vi "LV_n_UDP_clients.vi"() -> ()   [LabVIEW 2020]
panel:
  out "2nd port":string
  out "1st port":string
  in  "Open Multi Ports":bool
  in  "Open Single Port":bool
  in  "Send Test Image":bool
  in  "h":i32=10 min=1 max=5000 step=1
  in  "w":i32=1 min=1 max=5000 step=1
  out "Elaps ms":u32
  in  "Send Image":bool
  out "Path to Python script":path
  in  "Stop":bool
  out "Answer":string
  in  "Ping":bool
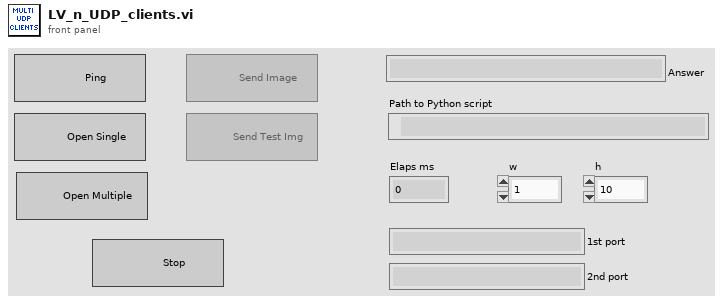
[diagram p1: front panel]
types:
  T1 = enum8{"Enabled", "Disabled", "Disabled and Grayed Out"}
  T2 = typedef "Image Type" = u32
  T3 = typedef "IMAQ Image.ctl" = refnum<image>
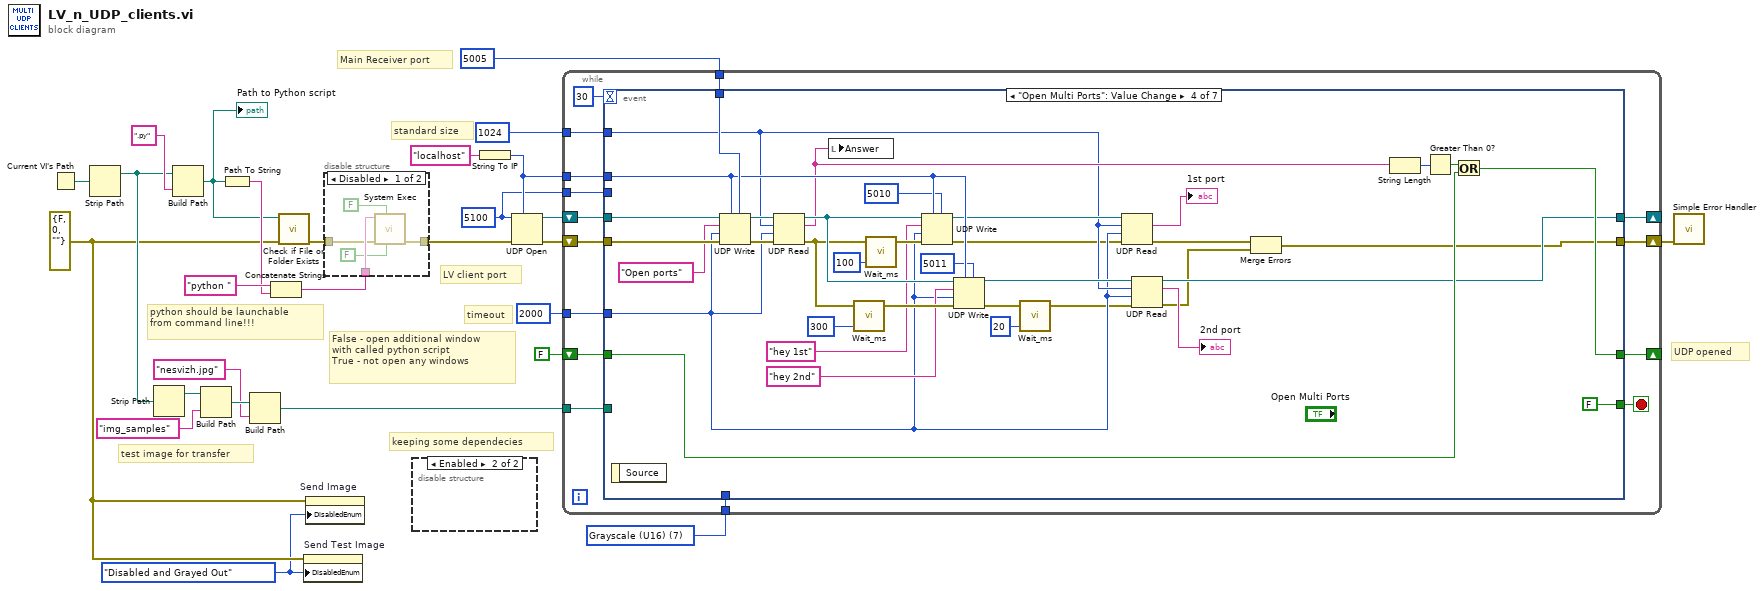
[diagram p0: block diagram]
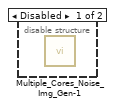
[diagram p2: hidden frame]
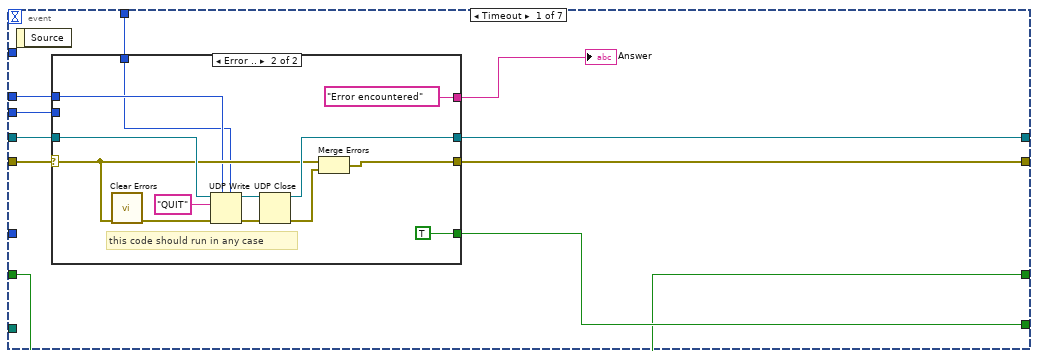
[diagram p4: hidden frame]
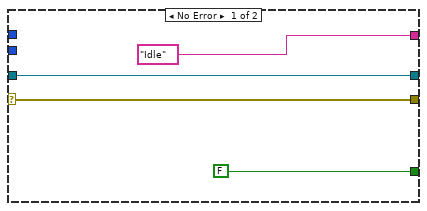
[diagram p5: hidden frame]
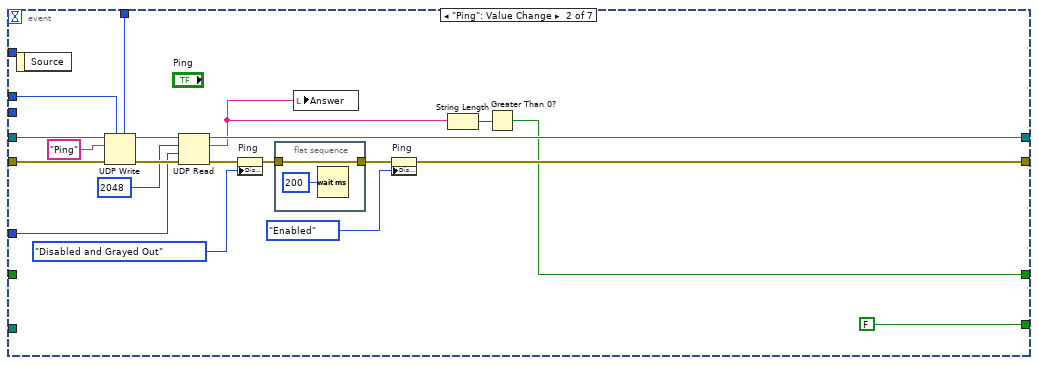
[diagram p6: hidden frame]
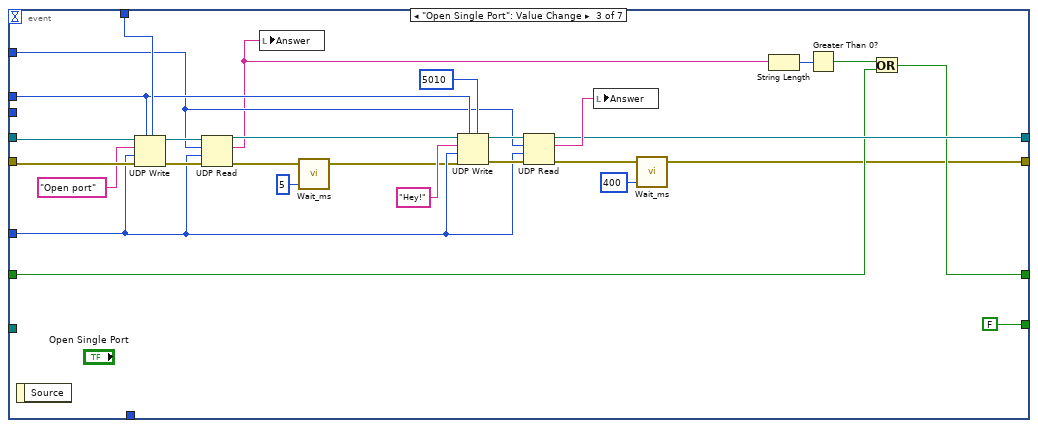
[diagram p7: hidden frame]
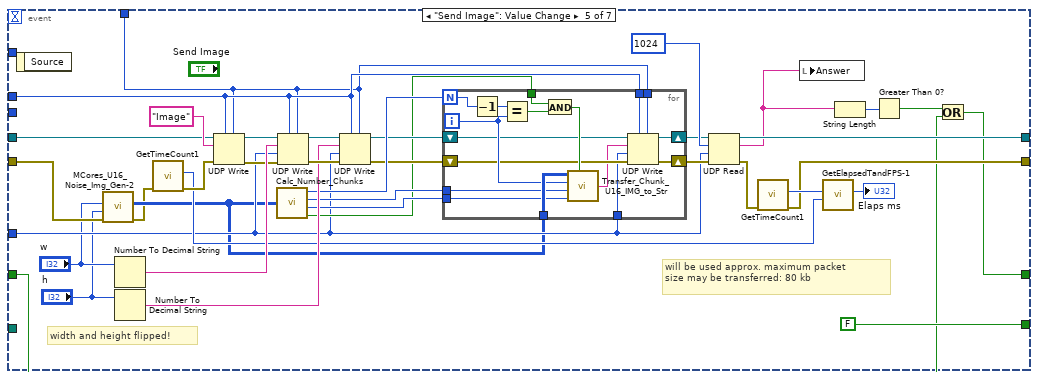
[diagram p8: hidden frame]
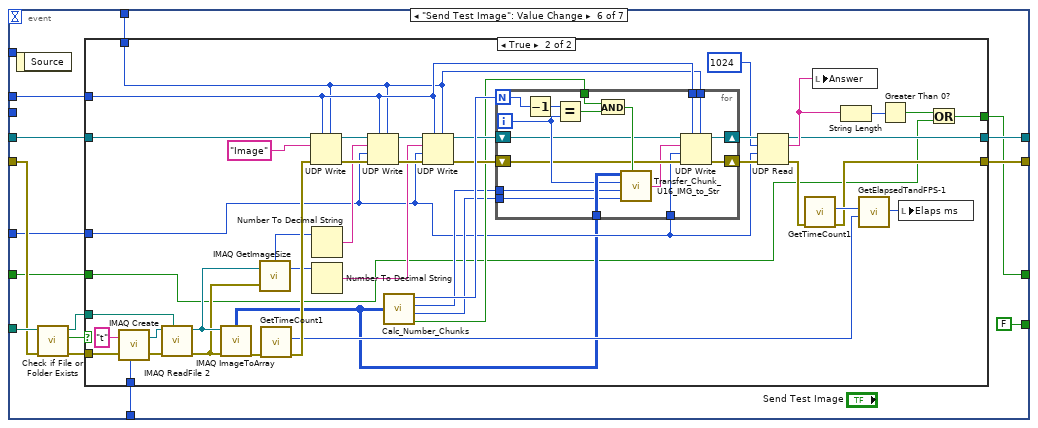
[diagram p9: hidden frame]
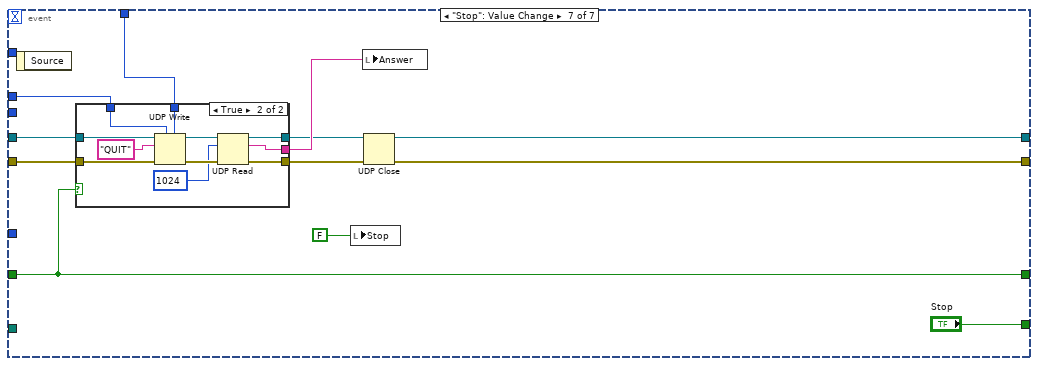
[diagram p11: hidden frame]
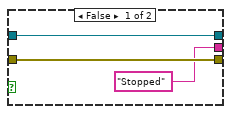
[diagram p12: hidden frame]
diagram:
  w3 = T1."Disabled and Grayed Out" ("Disabled")
  w5 = T2 7 items=["Grayscale (U8)", "Grayscale (I16)", "Grayscale (SGL)", "Complex (CSG)", "RGB (U32)", "HSL (U32)", "RGB (U64)", "Grayscale (U16)"] ("Image Type")
  w14 = u16 5100 ("remote port or service name")
  w4 = errorcluster {"status"=FALSE, "code"=0, "source"=""} ("error in (no error)")
  # "standard size"
  # "UDP opened"
  # "test image for transfer"
  # "keeping some dependecies"
  # "timeout"
  # "Main Receiver port"
  # "LV client port"
  # "False - open additional window\nwith called python script\nTrue - not open any windows"
  # "python should be launchable \nfrom command line!!!"
  n1 = Current VI's Path() -> (path=w26:path)
  n2 = Strip Path(path=w26) -> (stripped path=w11:path)  [unwired: 1 out]
  n3 = Strip Path(path=w11) -> (stripped path=w10:path)  [unwired: 1 out]
  n4 = Build Path(base path=w11, name or relative path=".py" ("string")) -> (appended path=w21:path)
  "Path to Python script" <- w21
  n5 = Build Path(base path=w10, name or relative path="img_samples" ("string")) -> (appended path=w8:path)
  n6 = Path To String(path=w21) -> (string=w22:string)
  n7 = Build Path(base path=w8, name or relative path="nesvizh.jpg" ("string")) -> (appended path=w6:path)
  n8 = Concatenate Strings("python " ("command line"), w22) -> (w24:string)
  n9 = call <vilib>:"Check if File or Folder Exists.vi"("error in (no error)"=w4, "path"=w21) -> ("error out"=w20:errorcluster)  [unwired: 7 in, 2 out]
  n10 = property on="Send Test Image" class="Bool"(error in=w4, "DisabledEnum"=w3) -> ()  [unwired: 1 in, 2 out]
  n11 = property on="Send Image" class="Bool"(error in=w4, "DisabledEnum"=w3) -> ()  [unwired: 1 in, 2 out]
  n12 = disable-structure shown="Disabled" {
    disable-tunnel: w24 -> [w32 _]
    disable-tunnel: [w31 w33] -> w19
    disable-tunnel: w20 -> [w29 w33]
    frame Disabled {
      n13 = call <vilib>:"System Exec.vi"("run minimized? (F)"=FALSE, "wait until completion? (T)"=FALSE, "error in (no error)"=w29, "command line"=w32) -> ("error out"=w31:errorcluster)  [unwired: 4 in, 3 out]
    }
    frame Enabled {
    }
  }
  n14 = disable-structure shown="Enabled" {
    frame Disabled {
      n15 = call "Multiple_Cores_Noise_Img_Gen-1.vi"() -> ()  [unwired: 10 in, 2 out]
    }
    frame Enabled {
    }
  }
  n16 = String To IP(1:"localhost" ("address")) -> (0:w15:u32)
  n17 = UDP Open(7:w15, 8:w19, 11:w14) -> (port=w17:refnum<k16>, 0:w18:errorcluster)  [unwired: 2 in, 1 out]
  n18 = while {
    shift-right: [w45] -> _
    shift-left: w17 -> [w46]
    shift-right: [w43] -> w27
    shift-left: w18 -> [w47]
    tunnel: w15 -> [w41]
    tunnel: w14 -> [w42]
    tunnel: u16 5005 ("remote port or service name") -> [w40]
    tunnel: 2000 -> [w39]
    tunnel: w6 -> [w38]
    tunnel: w5 -> [w37]
    shift-right: [w35] -> _
    shift-left: FALSE -> [w36]
    tunnel: 1024 -> [w34]
    stop <- w44 stop-if-true
    n19 = event shown="[3] \"Open Multi Ports\": Value Change" {
      selector: _ -> [_ _ _ _ _ _ _]
      dyn-events: _ -> [_ _ _ _ _ _ _]
      timeout: 30 -> [_ _ _ _ _ _ _]
      tunnel: [w54 FALSE ("Stop") FALSE ("Stop") FALSE ("Stop") FALSE ("Stop") FALSE ("Stop") "Stop"] -> w44
      tunnel: w47 -> [w58 w89 w125 w162 w172 w230 w303]
      tunnel: w46 -> [w57 w88 w124 w160 w199 w225 w304]
      tunnel: [w56 w84 w110 w134 w193 w220 w305] -> w45
      tunnel: [w55 w91 w99 w132 w185 w221 w306] -> w43
      tunnel: w42 -> [w52 _ _ _ _ _ _]
      tunnel: w41 -> [w51 w81 w118 w149 w174 w224 w299]
      tunnel: w40 -> [w50 w80 w122 w159 w173 w223 w298]
      tunnel: w39 -> [_ w79 w113 w130 w175 w222 _]
      tunnel: w38 -> [_ _ _ _ _ w231 _]
      tunnel: w37 -> [_ _ _ _ _ w226 _]
      tunnel: w36 -> [w49 _ w107 w142 w164 w218 w297]
      tunnel: [w49 w76 w105 w141 w163 w219 w297] -> w35
      tunnel: w34 -> [_ _ w112 w138 _ _ _]
      event Timeout {
        n20 = event-data() -> ()  [unwired: 1 in, 1 out]
        n21 = case shown="Error .." w58 {
          selector: w58 -> [w61 w70]
          tunnel: [w62 w73] -> w56
          tunnel: w57 -> [w62 w72]
          tunnel: [w61 w71] -> w55
          tunnel: [FALSE ("Stop") TRUE ("Stop")] -> w54
          tunnel: ["Idle" ("Answer") "Error encountered" ("Answer")] -> w53
          tunnel: w52 -> [_ _]
          tunnel: w51 -> [_ w69]
          tunnel: w50 -> [_ w68]
          frame No Error {
          }
          frame Error {
            # "this code should run in any case"
            n22 = call <vilib>:"Clear Errors.vi"("error in (no error)"=w70) -> ("error out"=w67:errorcluster)  [unwired: 5 in, 1 out]
            n23 = UDP Write(address=w69, port or service name=w68, connection ID=w72, data in="QUIT", 8:w67) -> (error out=w66:errorcluster, 3:w64:refnum<k16>)  [unwired: 1 in]
            n24 = UDP Close(connection ID=w64, 8:w66) -> (connection ID out=w73:refnum<k16>, error out=w63:errorcluster)
            n25 = Merge Errors(w70, w63) -> (w71:errorcluster)
          }
        }
        "Answer" <- w53
      }
      event "Ping": Value Change {
        n26 = event-data() -> ()  [unwired: 1 in, 1 out]
        n27 = UDP Write(address=w81, port or service name=w80, connection ID=w88, data in="Ping", 8:w89) -> (error out=w86:errorcluster, 3:w85:refnum<k16>)  [unwired: 1 in]
        n28 = UDP Read(connection ID=w85, max size (548)=2048 ("bytes to read"), timeout ms (25000)=w79, 8:w86) -> (data out=w78:string, error out=w83:errorcluster, 3:w84:refnum<k16>)  [unwired: 2 out]
        n29 = property on="Ping" class="Bool"(error in=w83, "DisabledEnum"=T1."Disabled and Grayed Out" ("Disabled")) -> (error out=w94:errorcluster)  [unwired: 1 in, 1 out]
        n30 = flat-sequence {
          tunnel: w94 -> [w96]
          tunnel: [w96] -> w92
          frame #0 {
            n31 = Wait (ms)(milliseconds to wait=u32 200) -> ()  [unwired: 1 out]
          }
        }
        n32 = local write "Answer"(w78) -> ()
        n33 = property on="Ping" class="Bool"(error in=w92, "DisabledEnum"=T1."Enabled" ("Disabled")) -> (error out=w91:errorcluster)  [unwired: 1 in, 1 out]
        n34 = String Length(string=w78) -> (length=w77:i32)
        n35 = Greater Than 0?(x=w77) -> (x > 0?=w76:bool)
      }
      event "Open Single Port": Value Change {
        n36 = event-data() -> ()  [unwired: 1 in, 1 out]
        n37 = UDP Write(address=w118, port or service name=w122, connection ID=w124, data in="Open port", 8:w125, 9:w113) -> (error out=w120:errorcluster, 3:w121:refnum<k16>)
        n38 = UDP Read(connection ID=w121, max size (548)=w112, timeout ms (25000)=w113, 8:w120) -> (data out=w108:string, error out=w103:errorcluster, 3:w119:refnum<k16>)  [unwired: 2 out]
        n39 = local write "Answer"(w108) -> ()
        n40 = call "Wait_ms.vi"("[IN] Suspend ms"=u32 5, "error IN"=w103) -> ("error OUT"=w102:errorcluster)  [unwired: 3 in]
        n41 = UDP Write(address=w118, port or service name=u16 5010, connection ID=w119, data in="Hey!", 8:w102, 9:w113) -> (error out=w114:errorcluster, 3:w115:refnum<k16>)
        n42 = UDP Read(connection ID=w115, max size (548)=w112, timeout ms (25000)=w113, 8:w114) -> (data out=w111:string, error out=w100:errorcluster, 3:w110:refnum<k16>)  [unwired: 2 out]
        n43 = local write "Answer"(w111) -> ()
        n44 = call "Wait_ms.vi"("[IN] Suspend ms"=u32 400, "error IN"=w100) -> ("error OUT"=w99:errorcluster)  [unwired: 3 in]
        n45 = String Length(string=w108) -> (length=w109:i32)
        n46 = Greater Than 0?(x=w109) -> (x > 0?=w106:bool)
        n47 = Or(x=w106, y=w107) -> (x .or. y?=w105:bool)
      }
      event "Open Multi Ports": Value Change {
        n48 = event-data() -> ()  [unwired: 1 in, 1 out]
        n49 = UDP Write(address=w149, port or service name=w159, connection ID=w160, data in="Open ports", 8:w162, 9:w130) -> (error out=w158:errorcluster, 3:w157:refnum<k16>)
        n50 = UDP Read(connection ID=w157, max size (548)=w138, timeout ms (25000)=w130, 8:w158) -> (data out=w143:string, error out=w151:errorcluster, 3:w153:refnum<k16>)  [unwired: 2 out]
        n51 = local write "Answer"(w143) -> ()
        n52 = call "Wait_ms.vi"("[IN] Suspend ms"=u32 300, "error IN"=w151) -> ("error OUT"=w150:errorcluster)  [unwired: 3 in]
        n53 = call "Wait_ms.vi"("[IN] Suspend ms"=u32 100, "error IN"=w151) -> ("error OUT"=w154:errorcluster)  [unwired: 3 in]
        n54 = UDP Write(address=w149, port or service name=u16 5010, connection ID=w153, data in="hey 1st", 8:w154, 9:w130) -> (error out=w127:errorcluster, 3:w140:refnum<k16>)
        n55 = UDP Write(address=w149, port or service name=u16 5011, connection ID=w153, data in="hey 2nd", 8:w150, 9:w130) -> (error out=w129:errorcluster, 3:w139:refnum<k16>)
        n56 = call "Wait_ms.vi"("[IN] Suspend ms"=u32 20, "error IN"=w129) -> ("error OUT"=w128:errorcluster)  [unwired: 3 in]
        n57 = UDP Read(connection ID=w140, max size (548)=w138, timeout ms (25000)=w130, 8:w127) -> (data out=→"1st port":string, error out=w135:errorcluster)  [unwired: 3 out]
        n58 = UDP Read(connection ID=w139, max size (548)=w138, timeout ms (25000)=w130, 8:w128) -> (data out=→"2nd port":string, error out=w133:errorcluster, 3:w134:refnum<k16>)  [unwired: 2 out]
        n59 = Merge Errors(w135, w133) -> (w132:errorcluster)
        n60 = String Length(string=w143) -> (length=w145:i32)
        n61 = Greater Than 0?(x=w145) -> (x > 0?=w144:bool)
        n62 = Or(x=w144, y=w142) -> (x .or. y?=w141:bool)
      }
      event "Send Image": Value Change {
        # "width and height flipped!"
        # "will be used approx. maximum packet \nsize may be transferred: 80 kb"
        n63 = event-data() -> ()  [unwired: 1 in, 1 out]
        n64 = call "MCores_U16_Noise_Img_Gen-2.vi"("error IN"=w172, "[IN] Width"="h", "[IN] Height"="w") -> ("error OUT"=w170:errorcluster, "[OUT] U16 Pixel Img"=w171:u16[][])  [unwired: 7 in]
        n65 = Number To Decimal String(number="w") -> (decimal integer string=w195:string)  [unwired: 1 in]
        n66 = Number To Decimal String(number="h") -> (decimal integer string=w192:string)  [unwired: 1 in]
        n67 = call "GetTimeCount1.vi"("error IN"=w170) -> ("error OUT"=w189:errorcluster, "[OUT] Timer Count"=w186:u32)  [unwired: 9 in]
        n68 = UDP Write(address=w174, port or service name=w173, connection ID=w199, data in="Image", 8:w189) -> (error out=w190:errorcluster, 3:w191:refnum<k16>)  [unwired: 1 in]
        n69 = call "Calc_Number_Chunks.vi"("[IN] U16 Pixel Img"=w171) -> ("[OUT] Number of chunks"=w182:i32, "[OUT] # rows single transfer"=w181:i32, "[OUT] # rows last transfer"=w180:i32, "[OUT] Not-equal last transfer"=w176:bool)
        n70 = UDP Write(address=w174, port or service name=w173, connection ID=w191, data in=w195, 8:w190, 9:w175) -> (error out=w198:errorcluster, 3:w197:refnum<k16>)
        n71 = UDP Write(address=w174, port or service name=w173, connection ID=w197, data in=w192, 8:w198, 9:w175) -> (error out=w178:errorcluster, 3:w179:refnum<k16>)
        n72 = for {
          N: w182 -> [w217]
          shift-right: [w207] -> w183
          shift-left: w178 -> [w208]
          tunnel: w171 -> [w215]
          tunnel: w181 -> [w210]
          tunnel: w180 -> [w209]
          shift-right: [w206] -> w177
          shift-left: w179 -> [w205]
          tunnel: w176 -> [w212]
          tunnel: w175 -> [w203]
          tunnel: w174 -> [w202]
          tunnel: w173 -> [w201]
          i -> [w213]
          n73 = Decrement(x=w217) -> (x-1=w216:i32)
          n74 = Equal?(x=w216, y=w213) -> (x = y?=w211:bool)
          n75 = And(x=w212, y=w211) -> (x .and. y?=w214:bool)
          n76 = call "Transfer_Chunk_U16_IMG_to_Str.vi"("[IN] U16 Pixel Img"=w215, "[IN] # of chunk"=w213, "[IN] # rows single transfer"=w210, "[IN] # rows last transfer"=w209, "[IN] Use remained rows"=w214) -> ("[OUT] Converted String"=w204:string)
          n77 = UDP Write(address=w202, port or service name=w201, connection ID=w205, data in=w204, 8:w208, 9:w203) -> (error out=w207:errorcluster, 3:w206:refnum<k16>)
        }
        n78 = UDP Read(connection ID=w177, max size (548)=1024 ("bytes to read"), timeout ms (25000)=w175, 8:w183) -> (data out=w166:string, error out=w188:errorcluster, 3:w193:refnum<k16>)  [unwired: 2 out]
        n79 = call "GetTimeCount1.vi"("error IN"=w188) -> ("error OUT"=w185:errorcluster, "[OUT] Timer Count"=w187:u32)  [unwired: 9 in]
        n80 = local write "Answer"(w166) -> ()
        n81 = call "GetElapsedTandFPS-1.vi"("[IN] Timer Count Before ALL [ms]"=w186, "[IN] Timer Count After ALL [ms]"=w187) -> ("[OUT] Elapsed time [ms]"=→"Elaps ms":u32)  [unwired: 3 in, 2 out]
        n82 = String Length(string=w166) -> (length=w167:i32)
        n83 = Greater Than 0?(x=w167) -> (x > 0?=w165:bool)
        n84 = Or(x=w165, y=w164) -> (x .or. y?=w163:bool)
      }
      event "Send Test Image": Value Change {
        n85 = event-data() -> ()  [unwired: 1 in, 1 out]
        n86 = call <vilib>:"Check if File or Folder Exists.vi"("error in (no error)"=w230, "path"=w231) -> ("error out"=w229:errorcluster, "file or folder exists?"=w228:bool, "dup path"=w227:path)  [unwired: 7 in]
        n87 = case shown="True" w228 {
          tunnel: w229 -> [w234 w279]
          tunnel: w227 -> [_ w274]
          tunnel: w226 -> [_ w278]
          tunnel: w225 -> [w235 w272]
          tunnel: w224 -> [_ w253]
          tunnel: w223 -> [_ w252]
          tunnel: w222 -> [_ w249]
          tunnel: [w234 w243] -> w221
          tunnel: [w235 w238] -> w220
          tunnel: [w233 w237] -> w219
          tunnel: w218 -> [w233 w236]
          frame False {
          }
          frame True {
            n88 = call "IMAQ Create"("Image Name"="t", "Image Type"=w278, "error in (no error)"=w279) -> ("New Image"=w275:T3, "error out"=w276:errorcluster)  [unwired: 2 in]
            n89 = call "IMAQ ReadFile 2"("File Path"=w274, "error in (no error)"=w276, "Image"=w275) -> ("error out"=w268:errorcluster, "Image Out"=w269:T3)  [unwired: 4 in, 3 out]
            n90 = call "IMAQ ImageToArray"("error in (no error)"=w268, "Image"=w269) -> ("error out"=w273:errorcluster, "Image Pixels (U8)"=w242:u8[][])  [unwired: 2 in, 3 out]
            n91 = call "IMAQ GetImageSize"("Image"=w269, "error in (no error)"=w268) -> ("Y Resolution"=w266:i32, "X Resolution"=w267:i32)  [unwired: 2 in, 1 out]
            n92 = call "GetTimeCount1.vi"("error IN"=w273) -> ("error OUT"=w271:errorcluster, "[OUT] Timer Count"=w246:u32)  [unwired: 9 in]
            n93 = UDP Write(address=w253, port or service name=w252, connection ID=w272, data in="Image", 8:w271) -> (error out=w265:errorcluster, 3:w264:refnum<k16>)  [unwired: 1 in]
            n94 = Number To Decimal String(number=w267) -> (decimal integer string=w263:string)  [unwired: 1 in]
            n95 = Number To Decimal String(number=w266) -> (decimal integer string=w260:string)  [unwired: 1 in]
            n96 = UDP Write(address=w253, port or service name=w252, connection ID=w264, data in=w263, 8:w265, 9:w249) -> (error out=w261:errorcluster, 3:w262:refnum<k16>)
            n97 = call "Calc_Number_Chunks.vi"("[IN] U16 Pixel Img"=w242) -> ("[OUT] Number of chunks"=w259:i32, "[OUT] # rows single transfer"=w255:i32, "[OUT] # rows last transfer"=w254:i32, "[OUT] Not-equal last transfer"=w256:bool)
            n98 = UDP Write(address=w253, port or service name=w252, connection ID=w262, data in=w260, 8:w261, 9:w249) -> (error out=w257:errorcluster, 3:w258:refnum<k16>)
            n99 = for {
              N: w259 -> [w296]
              shift-right: [w286] -> w251
              shift-left: w257 -> [w287]
              tunnel: w242 -> [w294]
              tunnel: w255 -> [w289]
              tunnel: w254 -> [w288]
              shift-right: [w285] -> w250
              shift-left: w258 -> [w284]
              tunnel: w256 -> [w291]
              tunnel: w249 -> [w282]
              tunnel: w253 -> [w281]
              tunnel: w252 -> [w280]
              i -> [w292]
              n100 = Decrement(x=w296) -> (x-1=w295:i32)
              n101 = Equal?(x=w295, y=w292) -> (x = y?=w290:bool)
              n102 = And(x=w291, y=w290) -> (x .and. y?=w293:bool)
              n103 = call "Transfer_Chunk_U16_IMG_to_Str.vi"("[IN] U16 Pixel Img"=w294, "[IN] # of chunk"=w292, "[IN] # rows single transfer"=w289, "[IN] # rows last transfer"=w288, "[IN] Use remained rows"=w293) -> ("[OUT] Converted String"=w283:string)
              n104 = UDP Write(address=w281, port or service name=w280, connection ID=w284, data in=w283, 8:w287, 9:w282) -> (error out=w286:errorcluster, 3:w285:refnum<k16>)
            }
            n105 = UDP Read(connection ID=w250, max size (548)=1024 ("bytes to read"), timeout ms (25000)=w249, 8:w251) -> (data out=w240:string, error out=w248:errorcluster, 3:w238:refnum<k16>)  [unwired: 2 out]
            n106 = call "GetTimeCount1.vi"("error IN"=w248) -> ("error OUT"=w243:errorcluster, "[OUT] Timer Count"=w247:u32)  [unwired: 9 in]
            n107 = local write "Answer"(w240) -> ()
            n108 = String Length(string=w240) -> (length=w241:i32)
            n109 = call "GetElapsedTandFPS-1.vi"("[IN] Timer Count Before ALL [ms]"=w246, "[IN] Timer Count After ALL [ms]"=w247) -> ("[OUT] Elapsed time [ms]"=w244:u32)  [unwired: 3 in, 2 out]
            n110 = Greater Than 0?(x=w241) -> (x > 0?=w239:bool)
            n111 = local write "Elaps ms"(w244) -> ()
            n112 = Or(x=w239, y=w236) -> (x .or. y?=w237:bool)
          }
        }
      }
      event "Stop": Value Change {
        n113 = event-data() -> ()  [unwired: 1 in, 1 out]
        n114 = case shown="True" w297 {
          tunnel: w304 -> [w311 w322]
          tunnel: w303 -> [w310 w321]
          tunnel: [w310 w317] -> w302
          tunnel: ["Stopped" ("data out") w316] -> w301
          tunnel: [w311 w315] -> w300
          tunnel: w299 -> [_ w313]
          tunnel: w298 -> [_ w312]
          frame False {
          }
          frame True {
            n115 = UDP Write(address=w313, port or service name=w312, connection ID=w322, data in="QUIT", 8:w321) -> (error out=w318:errorcluster, 3:w319:refnum<k16>)  [unwired: 1 in]
            n116 = UDP Read(connection ID=w319, max size (548)=1024 ("bytes to read"), 8:w318) -> (data out=w316:string, error out=w317:errorcluster, 3:w315:refnum<k16>)  [unwired: 1 in, 2 out]
          }
        }
        n117 = local write "Stop"(FALSE ("Stop")) -> ()
        n118 = local write "Answer"(w301) -> ()
        n119 = UDP Close(connection ID=w300, 8:w302) -> (connection ID out=w305:refnum<k16>, error out=w306:errorcluster)
      }
    }
  }
  n120 = call <vilib>:"Simple Error Handler.vi"("error in (no error)"=w27) -> ()  [unwired: 4 in, 5 out]
